vi "v0.2_RPM_pto.vi"(4 "PA:13":u32=1, 6 "PA:12":u32=1, 8 "error in":errorcluster, 10 "RPM's":i32=10, 11 "VISA COM IN":refnum<visa-resource-name>) -> (0 "error out":errorcluster, 2 "PTO_out":dbl, 3 "VISA COM OUT":refnum<visa-resource-name>)   [LabVIEW 2011]
doc: "<B>Velocidad mediante PTO</B>\n\nCambia la velocidad de salida del sermotor controlandola mediante un tren de pulsos. Se obtiene una velocidad muy precisa, esta velocidad depende de los parámetros con los que se ha configurado el driver.\n\n<B>Velocidad</B> Velocidad del servomotor en RPM's\n<B>Parámetro 12</B> Valor del Parámetro 12 en el Driver. default 0.\n<B>Parámetro 13</B> Valor del Parámetro 13 en el Driver. default 0."
panel:
  # "Fijar Velocidad del motor a travez del control de Posición"
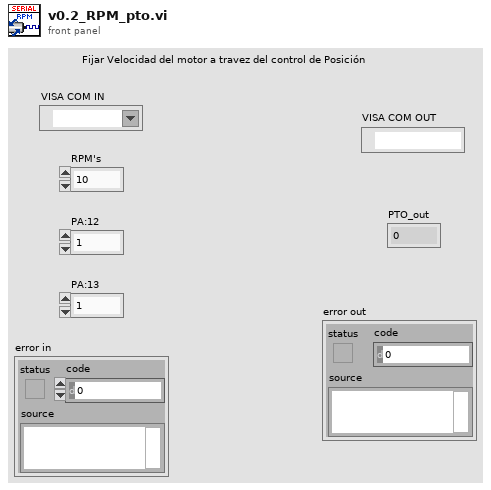
[diagram p1: front panel]
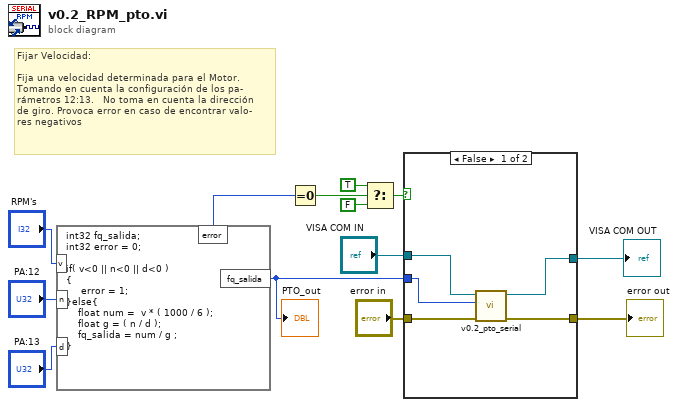
[diagram p0: block diagram]
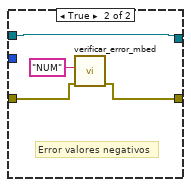
[diagram p2: hidden frame]
diagram:
  # "Fijar Velocidad:\n\nFija una velocidad determinada para el Motor.  \nTomando en cuenta la configuración de los pa-\nrámetros 12:13.   No toma en cuenta la dirección\nde giro. Provoca error en caso de encontrar valo-\nres negativos"
  n1 = formula code="int32 fq_salida;\nint32 error = 0;\n\nif( v<0 || n<0 || d<0 )\n{\n     error = 1; \n}else{\n    float num =  v * ( 1000 / 6 );\n    float g = ( n / d );\n    fq_salida = num / g ;\n}"("v"="RPM's", "n"="PA:12", "d"="PA:13") -> ("fq_salida"=w10:i32, "error"=w9:i32)
  "PTO_out" <- w10
  n2 = Equal To 0?(x=w9) -> (x = 0?=w8:bool)
  n3 = Select(t=TRUE, s=w8, f=FALSE) -> (s? t:f=w5:bool)
  n4 = case shown="False" w5 {
    tunnel: w10 -> [w18 _]
    tunnel: "error in" -> [w17 w21]
    tunnel: [w16 w20] -> w3
    tunnel: "VISA COM IN" -> [w15 w22]
    tunnel: [w14 w22] -> w1
    frame False {
      n5 = call "v0.2_pto_serial.vi"("error in (no error)"=w17, "Fout"=w18, "VISA COM IN"=w15) -> ("error out"=w16:errorcluster, "VISA COM OUT"=w14:refnum<visa-resource-name>)  [unwired: 7 in]
    }
    frame True {
      # "Error valores negativos"
      n6 = call "verificar_error_mbed.vi"("error in (no error)"=w21, "desde_mbed"="NUM") -> ("error out"=w20:errorcluster)  [unwired: 8 in, 1 out]
    }
  }
  "error out" <- w3
  "VISA COM OUT" <- w1
